vi "Mecanum Encoder.vi"() -> ()   [LabVIEW 2013]
panel:
  in  "counts/rev":dbl=240.0
  out "Wheel Speed R/sec":dbl format="%#_4g"
  out "Count":i32
  in  "Reset Counter":bool
  in  "Speed avg. #":dbl=6.0
  # "6"
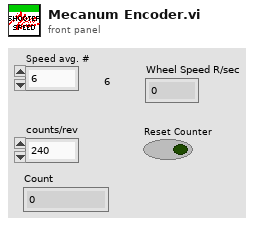
[diagram p1: front panel]
types:
  T1 = typedef "WPI_CounterDevRef.ctl" = cluster{"DevStatus":errorcluster, "CntIndex":T2}
  T2 = typedef "FPGA_CounterCtrSystemIndex.ctl" = enum8{"Ctr 0", "Ctr 1", "Ctr 2", "Ctr 3", "Ctr 4", "Ctr 5", "Ctr 6", "Ctr 7", "Invalid"}
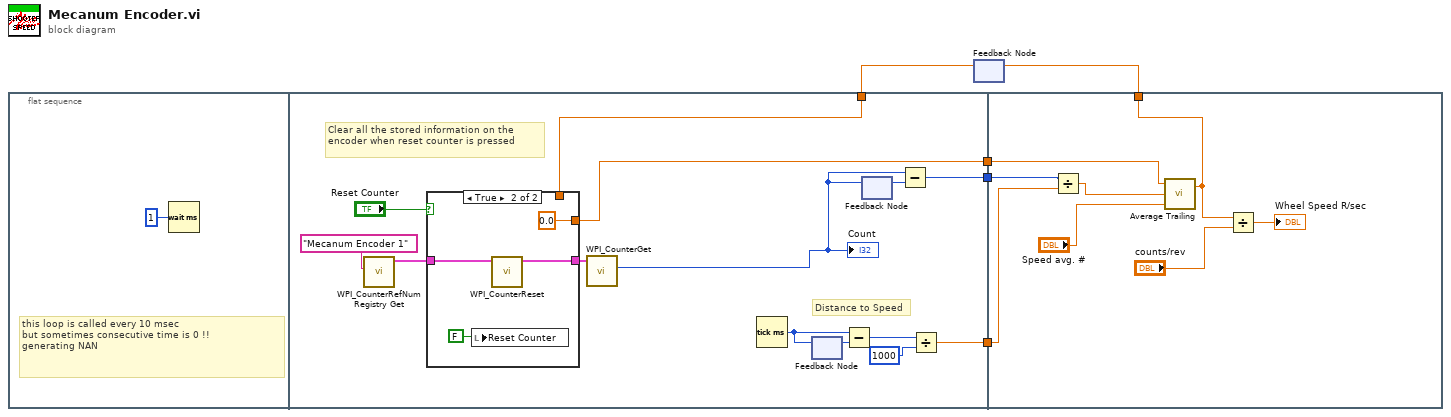
[diagram p0: block diagram]
diagram:
  n1 = flat-sequence {
    tunnel: [w10] -> w5
    tunnel: [w9] -> w4
    tunnel: [w8] -> w3
    tunnel: w1 -> [w7]
    tunnel: w5 -> [w31]
    tunnel: w4 -> [w29]
    tunnel: w3 -> [w30]
    tunnel: [w27] -> w2
    frame #0 {
      # "this loop is called every 10 msec\nbut sometimes consecutive time is 0 !!\ngenerating NAN"
      n2 = Wait (ms)(milliseconds to wait=u32 1) -> ()  [unwired: 1 out]
    }
    frame #1 {
      # "Distance to Speed"
      # "Clear all the stored information on the encoder when reset counter is pressed"
      n3 = call <vilib>:"WPI_CounterRefNum Registry Get.vi"("refnum name"="Mecanum Encoder 1") -> ("CounterDevRef"=w15:T1)  [unwired: 9 in, 1 out]
      n4 = case shown="True" "Reset Counter" {
        tunnel: w15 -> [w22 w25]
        tunnel: [w22 w24] -> w12
        tunnel: w7 -> [w21 _]
        tunnel: [w21 0.0 ("Output")] -> w8
        frame False {
        }
        frame True {
          n5 = local write "Reset Counter"(FALSE) -> ()
          n6 = call <vilib>:"WPI_CounterReset.vi"("CounterDevRef in"=w25) -> ("CounterDevRef out"=w24:T1)  [unwired: 9 in, 1 out]
        }
      }
      n7 = call <vilib>:"WPI_CounterGet.vi"("CounterDevRef in"=w12) -> ("Value"=w11:i32)  [unwired: 5 in, 5 out]
      "Count" <- w11
      n8 = Tick Count (ms)() -> (millisecond timer value=w16:u32)
      n9 = feedback #1() -> (w17:u32)  [unwired: 1 in]
      n10 = feedback-in #1(w16) -> ()
      n11 = Subtract(x=w16, y=w17) -> (x-y=w19:u32)
      n12 = feedback #2() -> (w20:i32)  [unwired: 1 in]
      n13 = feedback-in #2(w11) -> ()
      n14 = Subtract(x=w11, y=w20) -> (x-y=w10:i32)
      n15 = Divide(x=w19, y=u32 1000) -> (x/y=w9:dbl)
    }
    frame #2 {
      n16 = Divide(x=w31, y=w29) -> (x/y=w32:dbl)
      n17 = call "Average Trailing.vi"("averg #"="Speed avg. #", "Input"=w32, "Previous\nValue"=w30) -> ("Output"=w27:dbl)  [unwired: 1 in]
      n18 = Divide(x=w27, y="counts/rev") -> (x/y=→"Wheel Speed R/sec":dbl)
    }
  }
  n19 = feedback #3() -> (w1:dbl)  [unwired: 1 in]
  n20 = feedback-in #3(w2) -> ()
